vi "DP I-O Init Data File.vi"(0 "DP stimulus params":T2={"Ear"=enum."Right", "f2 freqs (kHz)"="5.6;8.0;11.3;16;22.6;32;", "Start (dB)"=20.0, "Stop (dB)"=70.0, "Step (dB)"=10.0, "Mode"=enum."L1 = L2 + 10 dB", "override recal"=FALSE, "Sampling Rate (Hz)"=0.0, "Frame (ms)"=0}, 5 "Sampling interval (us)":dbl, 7 "Averaging Specs":T3={"#Waves to Ave"=25, "#Spectra to Ave"=4}, 9 "NOTES":string, 11 "error in (no error)":errorcluster, 12 "Expt State":T1, 13 "Probe Mic Gain (dB)":dbl) -> (4 "Path":path, 14 "Expt State out":T1, 15 "error out":errorcluster)   [LabVIEW 2020]
uses:
  CFTS SubVIs/CFTS-Data Type Enum.ctl
  epl-vi-lib/Utility VIs/File IO VIs/Configuration File Wrapper VIs/Config-Read Key (string).vi
  Typedefs/DP Stimulus Params.ctl
  CFTS SubVIs/CFTS-Experiment State.ctl
panel:
  in  "Type of Run":string="DP I-O"
  in  "Acoustic System":u16(ring)=3 items=["", "ER-10c System", "", "Starship System"]
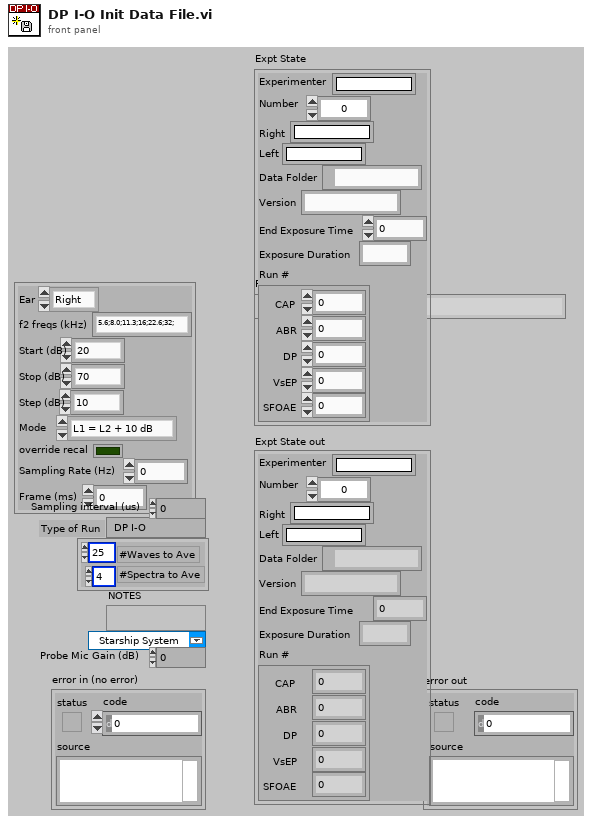
[diagram p1: front panel]
types:
  T1 = typedef "CFTS-Experiment State.ctl" = cluster{"Experimenter":string, "Number":u32, "Right":string, "Left":string, "Data Folder":path, "Version":string, "End Exposure Time":dbl, "Exposure Duration":string, "Run #":cluster{"CAP":i32, "ABR":i32, "DP":i32, "VsEP":i32, "SFOAE":i32}}
  T2 = typedef "DP Stimulus Params.ctl" = cluster{"Ear":enum16{"Right", "Left"}, "f2 freqs (kHz)":string, "Start (dB)":dbl, "Stop (dB)":dbl, "Step (dB)":dbl, "Mode":enum16{"L1 = L2", "L1 = L2 + 10 dB"}, "override recal":bool, "Sampling Rate (Hz)":dbl, "Frame (ms)":i32}
  T3 = cluster{"#Waves to Ave":i32, "#Spectra to Ave":i32}
  T4 = typedef "CFTS-Data Type Enum.ctl" = enum16{"CAP", "ABR", "DP", "VsEP", "MeasSeq", "SFOAE"}
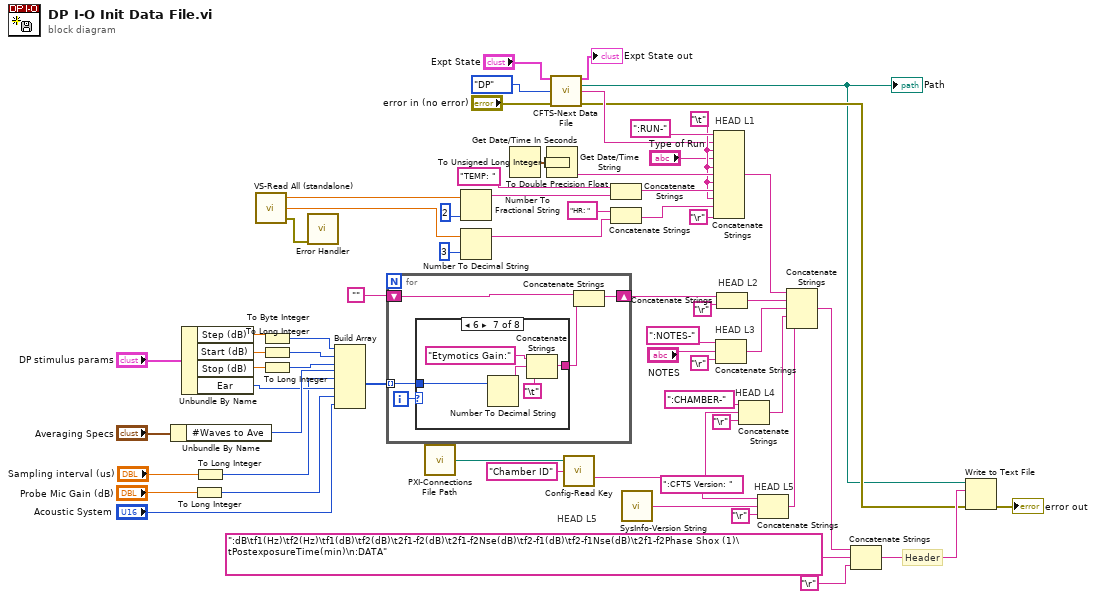
[diagram p0: block diagram]
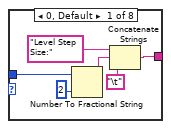
[diagram p2: hidden frame]
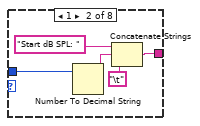
[diagram p3: hidden frame]
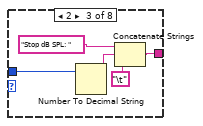
[diagram p4: hidden frame]
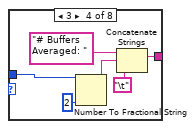
[diagram p5: hidden frame]
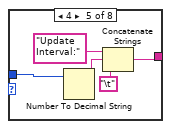
[diagram p6: hidden frame]
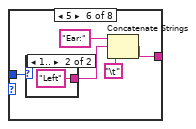
[diagram p7: hidden frame]
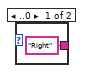
[diagram p8: hidden frame]
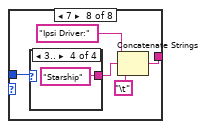
[diagram p9: hidden frame]
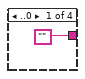
[diagram p10: hidden frame]
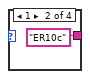
[diagram p11: hidden frame]
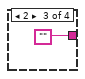
[diagram p12: hidden frame]
diagram:
  w48 = "\t"
  # "HEAD L5"
  # "HEAD L4"
  # "HEAD L1"
  # "Header"
  # "HEAD L5"
  # "HEAD L3"
  # "HEAD L2"
  n1 = Unbundle By Name("Averaging Specs") -> ("#Waves to Ave"=w33:i32)
  n2 = Unbundle By Name("DP stimulus params") -> ("Step (dB)"=w31:dbl, "Start (dB)"=w30:dbl, "Stop (dB)"=w29:dbl, "Ear"=w25:enum16{"Right", "Left"})
  n3 = To Long Integer(number="Probe Mic Gain (dB)") -> (32bit integer=w11:i32)
  n4 = To Long Integer(number="Sampling interval (us)") -> (32bit integer=w13:i32)
  n5 = call "VS-Read All (standalone).vi"() -> ("error out"=w4:errorcluster, "Heart Rate (bpm)"=w5:dbl, "Temperature (C)"=w6:dbl)  [unwired: 3 in]
  n6 = To Byte Integer(number=w31) -> (8bit integer=w28:i8)
  n7 = To Long Integer(number=w30) -> (32bit integer=w27:i32)
  n8 = To Long Integer(number=w29) -> (32bit integer=w26:i32)
  n9 = call "Error Handler.vi"("error in (no error)"=w4) -> ()  [unwired: 13 in, 2 out]
  n10 = Build Array(w28, w27, w26, w33, w13, w25, w11, "Acoustic System") -> (w54:i32[])
  n11 = for {
    shift-right: [w70] -> w63
    shift-left: "" -> [w71]
    tunnel: w54 -> [w68] mode=indexing
    i -> [w69]
    n12 = case shown="6" w69 {
      tunnel: w68 -> [w73 w78 w84 w89 w95 w100 w108 w111]
      tunnel: [w72 w79 w83 w88 w94 w99 w106 w112] -> w67
      frame 0, Default {
        n13 = Number To Fractional String(number=w73, precision (6)=2) -> (F-format string=w76:string)  [unwired: 2 in]
        n14 = Concatenate Strings("Level Step Size:", w76, "\t") -> (w72:string)
      }
      frame 1 {
        n15 = Number To Decimal String(number=w78) -> (decimal integer string=w81:string)  [unwired: 1 in]
        n16 = Concatenate Strings("Start dB SPL: ", w81, "\t") -> (w79:string)
      }
      frame 2 {
        n17 = Number To Decimal String(number=w84) -> (decimal integer string=w87:string)  [unwired: 1 in]
        n18 = Concatenate Strings("Stop dB SPL: ", w87, "\t") -> (w83:string)
      }
      frame 3 {
        n19 = Number To Fractional String(number=w89, precision (6)=2) -> (F-format string=w92:string)  [unwired: 2 in]
        n20 = Concatenate Strings("# Buffers Averaged: ", w92, "\t") -> (w88:string)
      }
      frame 4 {
        n21 = Number To Decimal String(number=w95) -> (decimal integer string=w97:string)  [unwired: 1 in]
        n22 = Concatenate Strings("Update Interval:", w97, "\t") -> (w94:string)
      }
      frame 5 {
        n23 = case shown="1.." w100 {
          tunnel: ["Right" "Left"] -> w103
          frame ..0 {
          }
          frame 1.. {
          }
        }
        n24 = Concatenate Strings("Ear:", w103, "\t") -> (w99:string)
      }
      frame 6 {
        n25 = Number To Decimal String(number=w108) -> (decimal integer string=w110:string)  [unwired: 1 in]
        n26 = Concatenate Strings("Etymotics Gain:", w110, "\t") -> (w106:string)
      }
      frame 7 {
        n27 = case shown="3.." w111 {
          tunnel: ["" "ER10c" "" "Starship"] -> w115
          frame ..0 {
          }
          frame 1 {
          }
          frame 2 {
          }
          frame 3.. {
          }
        }
        n28 = Concatenate Strings("Ipsi Driver:", w115, "\t") -> (w112:string)
      }
    }
    n29 = Concatenate Strings(w71, w67) -> (w70:string)
  }
  n30 = call "PXI-Connections File Path.vi"() -> ("Path"=w1:path)  [unwired: 1 in]
  n31 = Number To Fractional String(number=w6, precision (6)=2) -> (F-format string=w60:string)  [unwired: 2 in]
  n32 = Number To Decimal String(number=w5, width (-)=3) -> (decimal integer string=w45:string)
  n33 = Get Date/Time In Seconds() -> (seconds since 1Jan1904=w35:timestamp)
  n34 = To Double Precision Float(number=w35) -> (double precision float=w36:dbl)
  n35 = To Unsigned Long Integer(number=w36) -> (unsigned 32bit integer=w66:u32)
  n36 = Get Date/Time String(seconds (now)=w66) -> (time string=w64:string)  [unwired: 2 in, 1 out]
  n37 = call "CFTS-Next Data File.vi"("Expt State"="Expt State", "Data Type"=CFTS-Data_Type_Enum."DP", "error in (no error)"="error in (no error)") -> ("Expt State out"=→"Expt State out":T1, "Datafile path"=w18:path, "run #"=w23:string, "error out"=w22:errorcluster)  [unwired: 8 in, 1 out]
  "Path" <- w18
  n38 = call-poly "Config-Read Key.vi"("configuration file path"=w1, "key"="Chamber ID" ("string")) -> ("value"=w2:string)  [unwired: 10 in, 3 out]
  n39 = Concatenate Strings("TEMP: ", w60) -> (w59:string)
  n40 = Concatenate Strings("HR: ", w45) -> (w47:string)
  n41 = call "SysInfo-Version String.vi"() -> ("Version String"=w8:string)  [unwired: 1 in]
  n42 = Concatenate Strings(":RUN-", w23, w48, "Type of Run", w48, w64, w48, w59, w48, w47, "\r") -> (w58:string)
  n43 = Concatenate Strings(":NOTES-", "NOTES", "\r") -> (w53:string)
  n44 = Concatenate Strings(w63, "\r") -> (w57:string)
  n45 = Concatenate Strings(":CHAMBER-", w2, "\r") -> (w40:string)
  n46 = Concatenate Strings(":CFTS Version: ", w8, "\r") -> (w7:string)
  n47 = Concatenate Strings(w58, w57, w53, w40, w7) -> (w51:string)
  n48 = Concatenate Strings(w51, ":dB\tf1(Hz)\tf2(Hz)\tf1(dB)\tf2(dB)\t2f1-f2(dB)\t2f1-f2Nse(dB)\tf2-f1(dB)\tf2-f1Nse(dB)\t2f1-f2Phase Shox (1)\tPostexposureTime(min)\n:DATA", "\r") -> (w50:string)
  n49 = Write to Text File(file (use dialog)=w18, text=w50, error in=w22) -> (error out=→"error out":errorcluster)  [unwired: 1 in, 2 out]
